vi "equilibrium_measurements.vi"() -> ()   [LabVIEW 2019]
uses:
  <vilib>/userDefined/High Color/IMAQdx.ctl
  <vilib>/vision/driver/IMAQdx.llb/IMAQdx Attribute Type.ctl
  <vilib>/vision/Management.llb/Cast Image 2 Method.ctl
  <vilib>/DAQmx/write.llb/DAQmx Write (Analog DBL 1Chan 1Samp).vi
  <vilib>/DAQmx/read.llb/DAQmx Read (Analog DBL 1Chan 1Samp).vi
  <vilib>/Analysis/baseanly.llb/Mean (DBL).vi
  <vilib>/DAQmx/create/channels.llb/DAQmx Create Channel (AO-Voltage-Basic).vi
  <vilib>/DAQmx/miscellaneous.llb/DAQmx Fill In Error Info.vi
  <vilib>/DAQmx/create/channels.llb/DAQmx Create Channel (AI-Temperature-Thermocouple).vi
  <vilib>/vision/driver/NI_Vision_Acquisition_Software.lvlib
  <resource>/objmgr/imaqdx.rc
  <vilib>/vision/NI_Vision_Development_Module.lvlib
  <vilib>/Analysis/NI_AALBase.lvlib
panel:
  out "Video":bool
  in  "Action":i32(listbox)
  out "meanIntensity":dbl[](array[numeric])
  out "varLaplacian":dbl[](array[numeric])
  out "mean":dbl
  out "variance":dbl
  out "Avg Intensity":dbl(graph)=4.716017316017316
  in  "Activate":bool
  out "Var of Laplacian":dbl(graph)=63.940469067936796
  out "Camera Display 2":T1(plugin-control) caption="Image Out"
  in  "ROI":T2={"Global Rectangle"=[], "Contours"=[{"Contour Type"=0, "ROI Type"=3, "Points"=[231, 86, 235, 90]}, {"Contour Type"=0, "ROI Type"=3, "Points"=[193, 50, 270, 125]}]}
  in  "error in":errorcluster
  in  "File path for video":string="C:\\Users\\Aniket\\Desktop\\mCherry_calibration\\new_lens\\laser_calibration\\laser_and_heating\\"
  in  "Laser profile file path":path=path "C:/Users/Aniket/Desktop/mCherry_calibration/new_lens/laser_calibration/laser_profiles/new_profile.txt"
  in  "Trigger Laser":bool
  in  "Power Generator":refnum<visa-resource-name>="COM3"
  in  "Desired \nTemperature":dbl=20.0 format="%#_13g"
  in  "PID Control":bool
  in  "Image file path \n(Do not add specify file extension - set to png)":path=path "C:/Users/Aniket/Desktop/mCherry_calibration/new_lens/laser_calibration/laser_profiles.txt"
  out "Current \nTemperature":dbl format="%0.2f"
  out "?":dbl[](graph)=[37.63236695538445]
  out "error out 7":errorcluster
  out "error out 6":errorcluster
  out "error out 5":errorcluster
  out "Exposure Time":dbl
  in  "ON/OFF":bool
  out "error out 3":errorcluster
  in  "LED":dbl(slide) scale=0.0..10.0
  in  "Refresh":bool
  out "Record":bool
  out "Processed Frames per Second":dbl
  out "Acquired Frame Rate":dbl
  out "error out":errorcluster
  out "Camera Display":T1(plugin-control) caption="Image Out"
  in  "Frame Rate":dbl=20.0
  out "Attribute Information Array":T4(array[cluster])
  in  "Session In":T5="cam0"
  # "Spot motion"
  # "Stage motion"
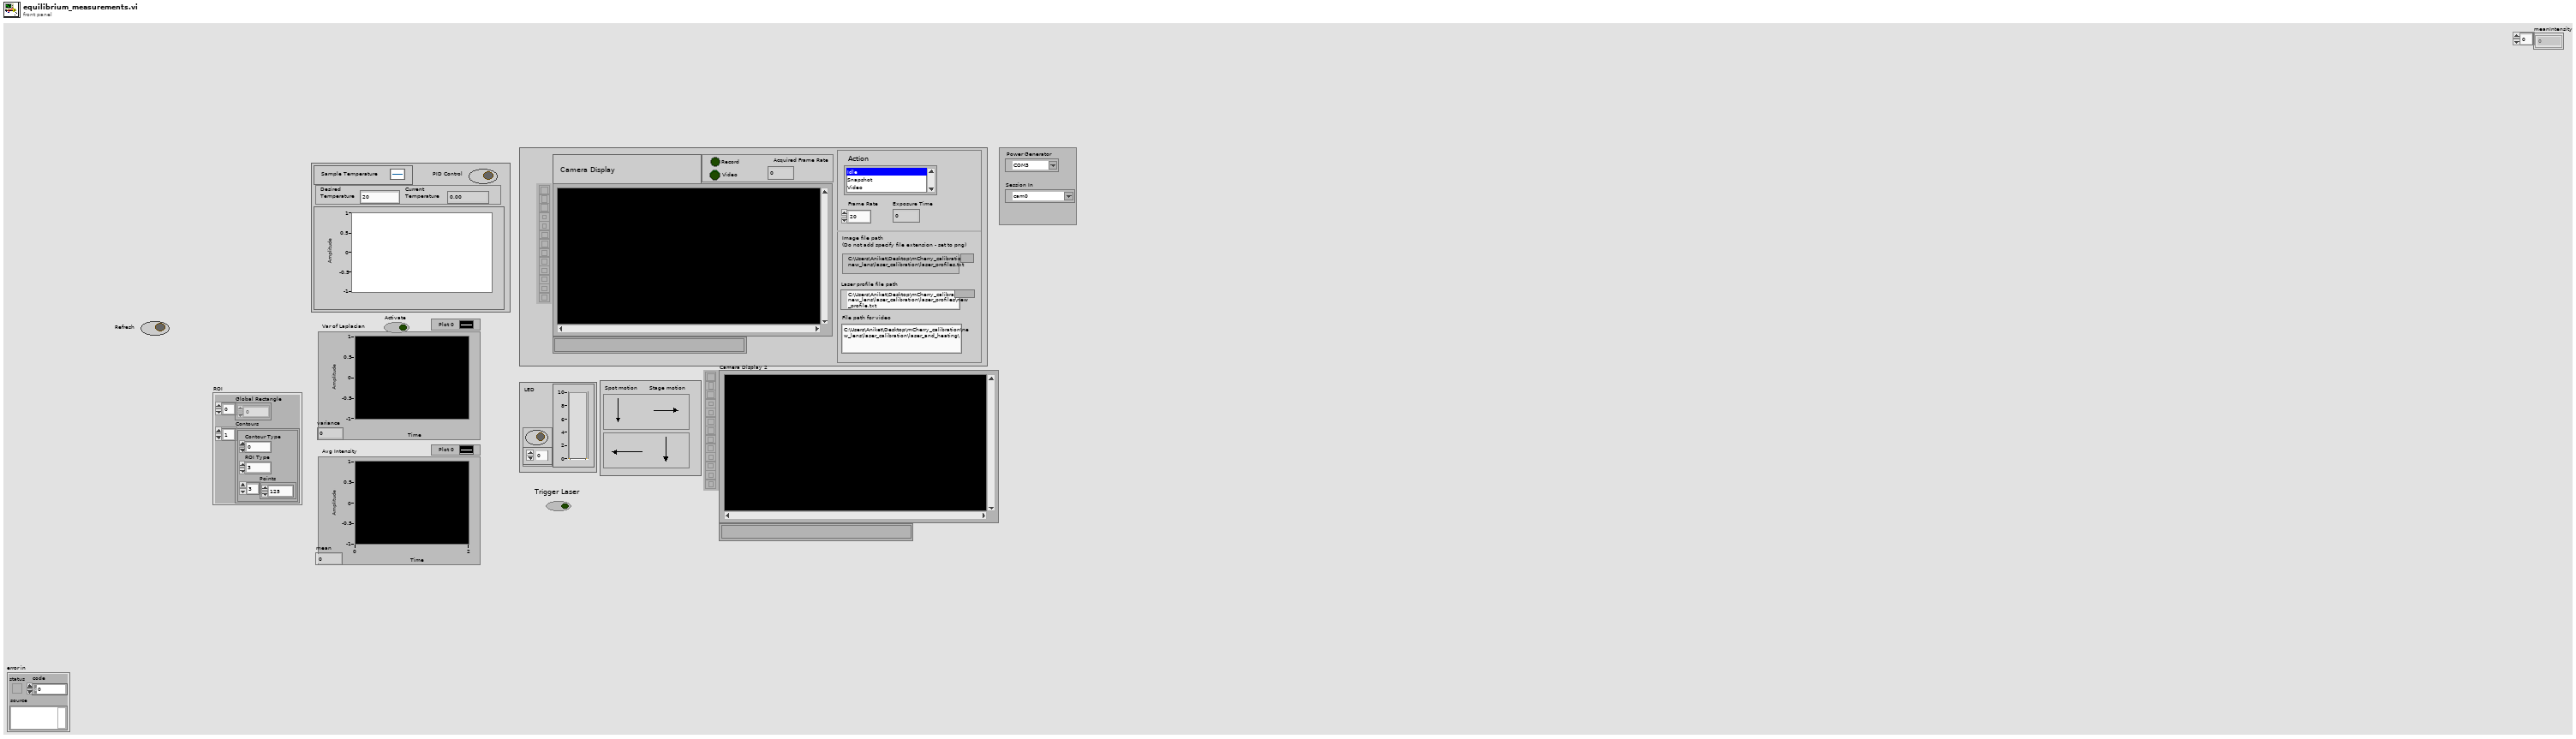
[diagram p1: front panel]
types:
  T1 = typedef "IMAQ Image.ctl" = refnum<image>
  T2 = cluster{"Global Rectangle":i32[], "Contours":cluster{"Contour Type":u32, "ROI Type":u32, "Points":i32[]}[]}
  T3 = typedef "NI_Vision_Acquisition_Software.lvlib/IMAQdx Attribute Type.ctl" = enum32{"U32", "I64", "DBL", "String", "Enum", "Bool", "Command"}
  T4 = cluster{"Attribute Type":T3, "Readable":bool, "Writable":bool, "Attribute Name":string}[]
  T5 = typedef "IMAQdx.ctl" = refnum<k21>
  T6 = typedef "Image Type" = u32
  T7 = typedef "ROI Descriptor" = cluster{"Global Rectangle":i32[], "Contours":cluster{"ID":enum32{"External", "Internal"}, "Type":u32, "Coordinates":i32[]}[]}
  T8 = typedef "IMAQ Rectangle" = cluster{"Left":i32, "Top":i32, "Right":i32, "Bottom":i32, "Rotation":dbl}
  T9 = typedef "Cast Image 2 Method.ctl" = u32
  T10 = typedef "IMAQ AVI2 Refnum.ctl" = refnum<k20>
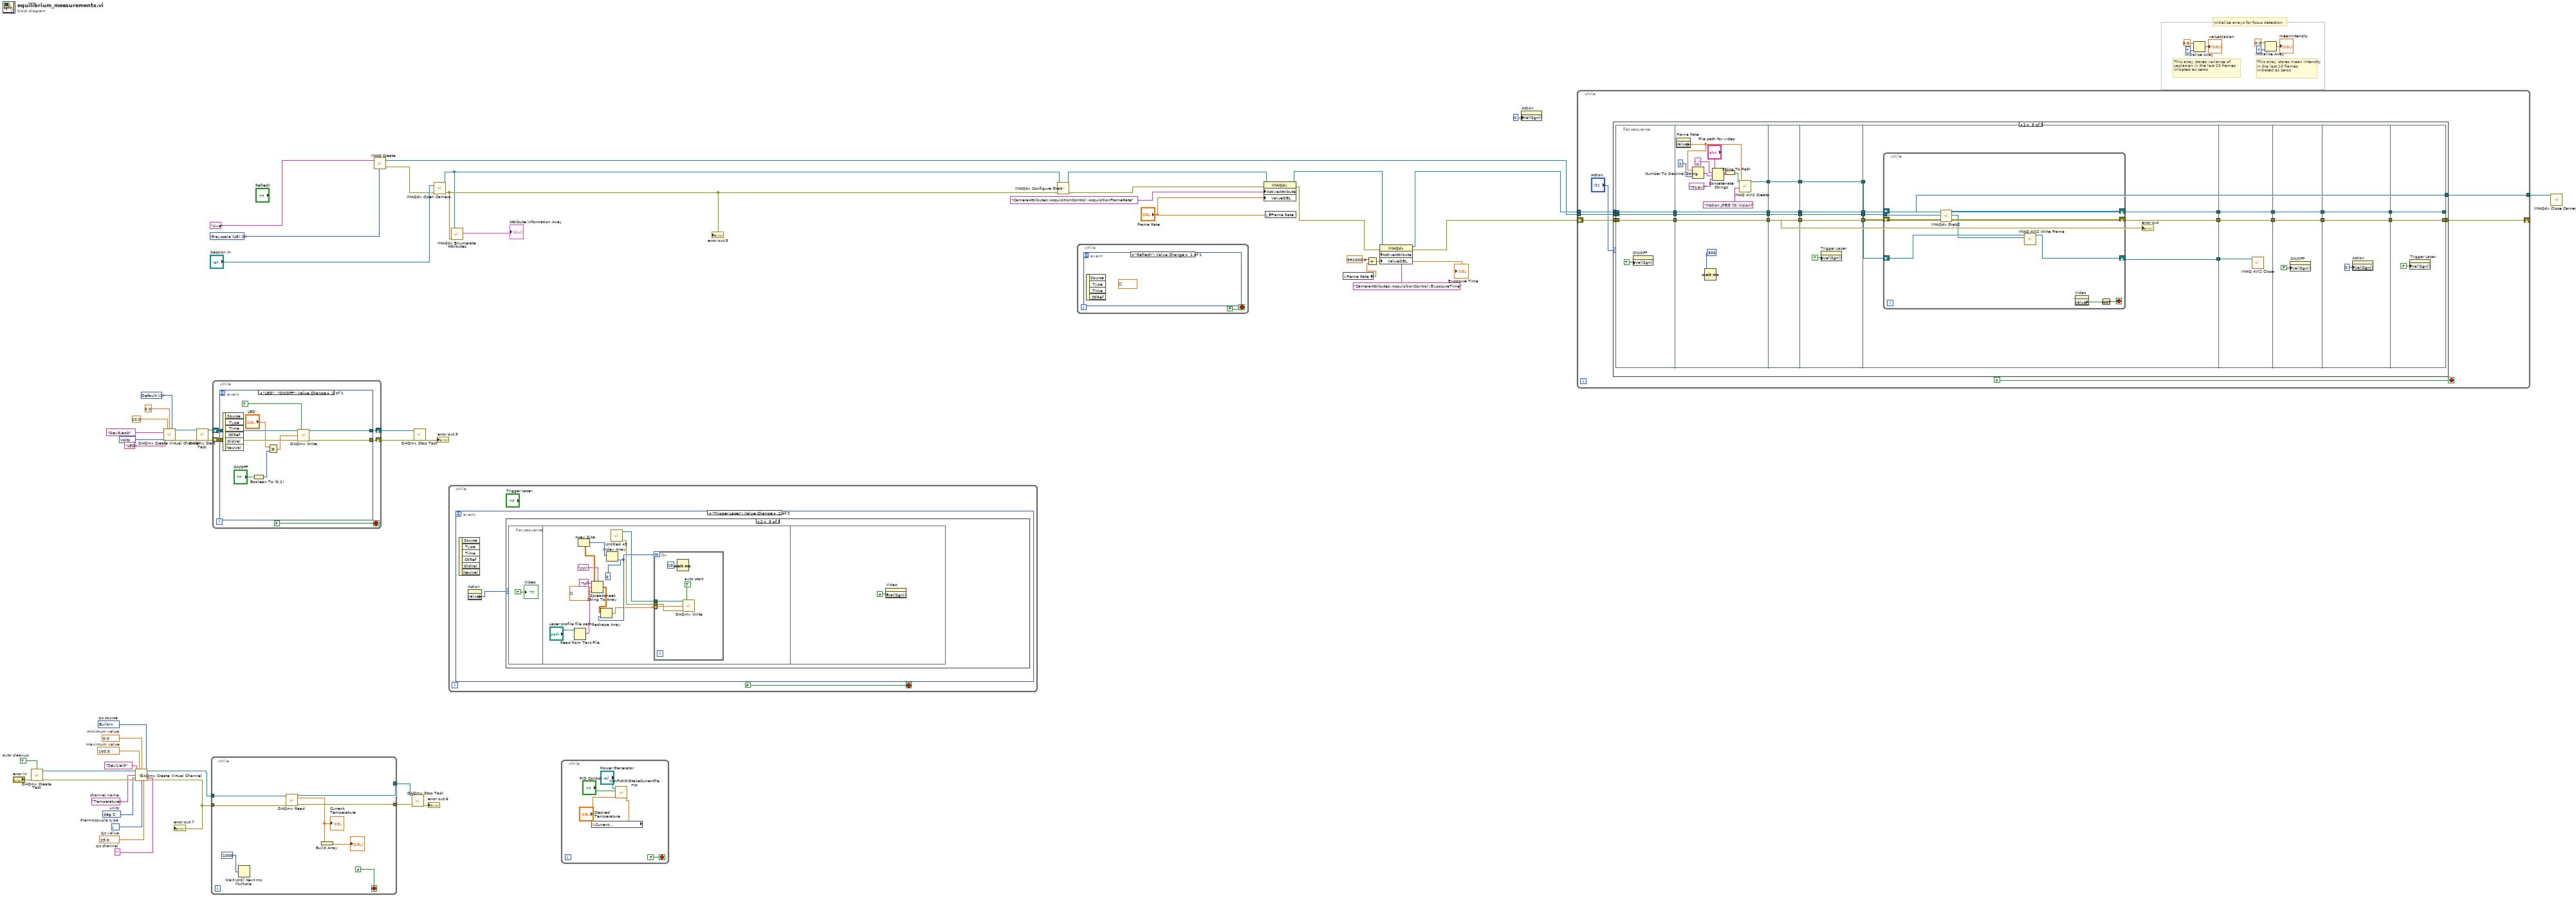
[diagram p0: block diagram]
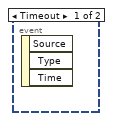
[diagram p2: hidden frame]
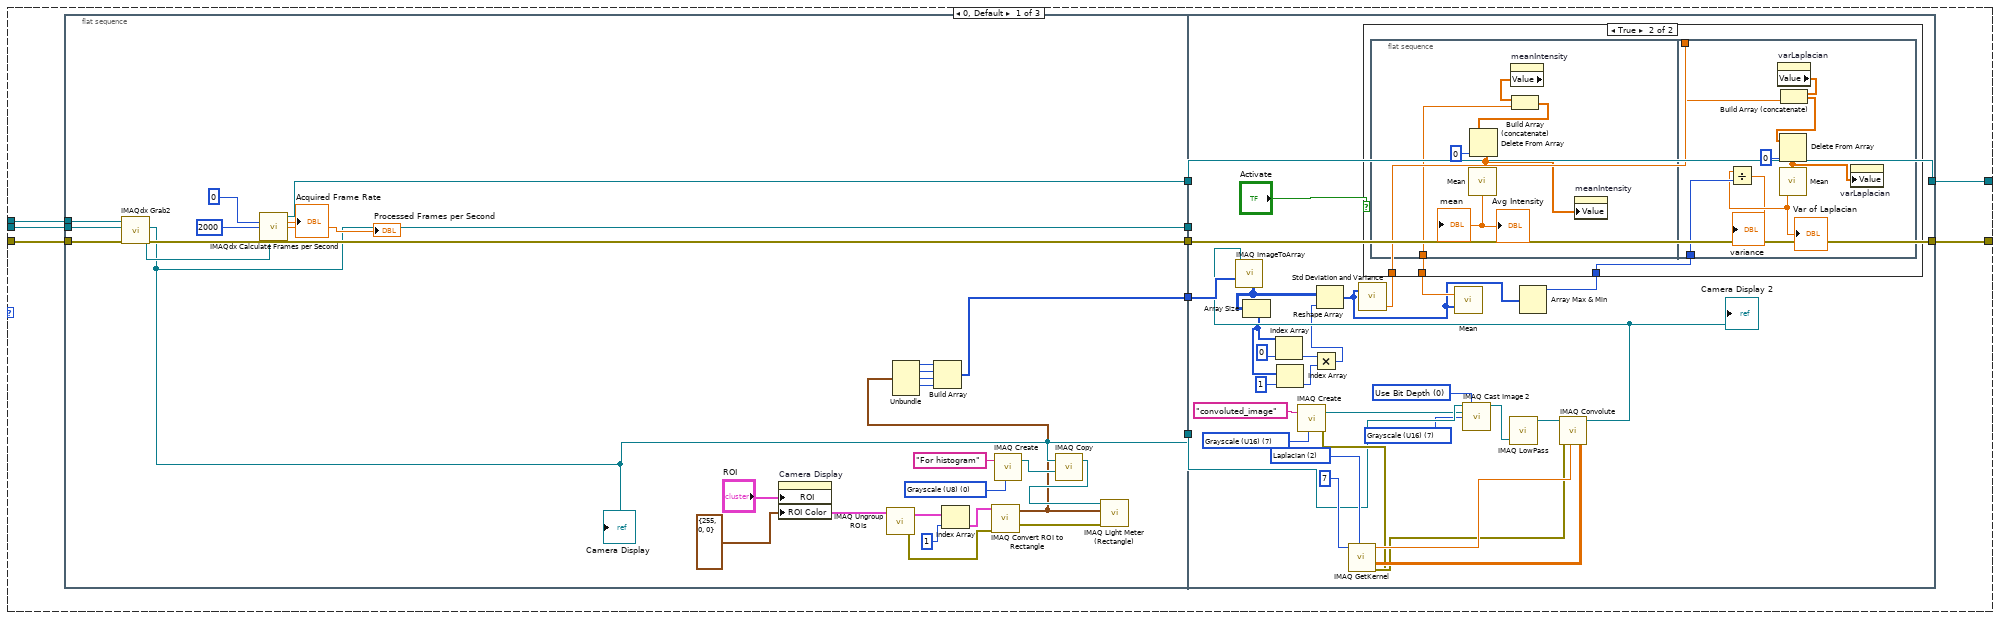
[diagram p5: hidden frame]
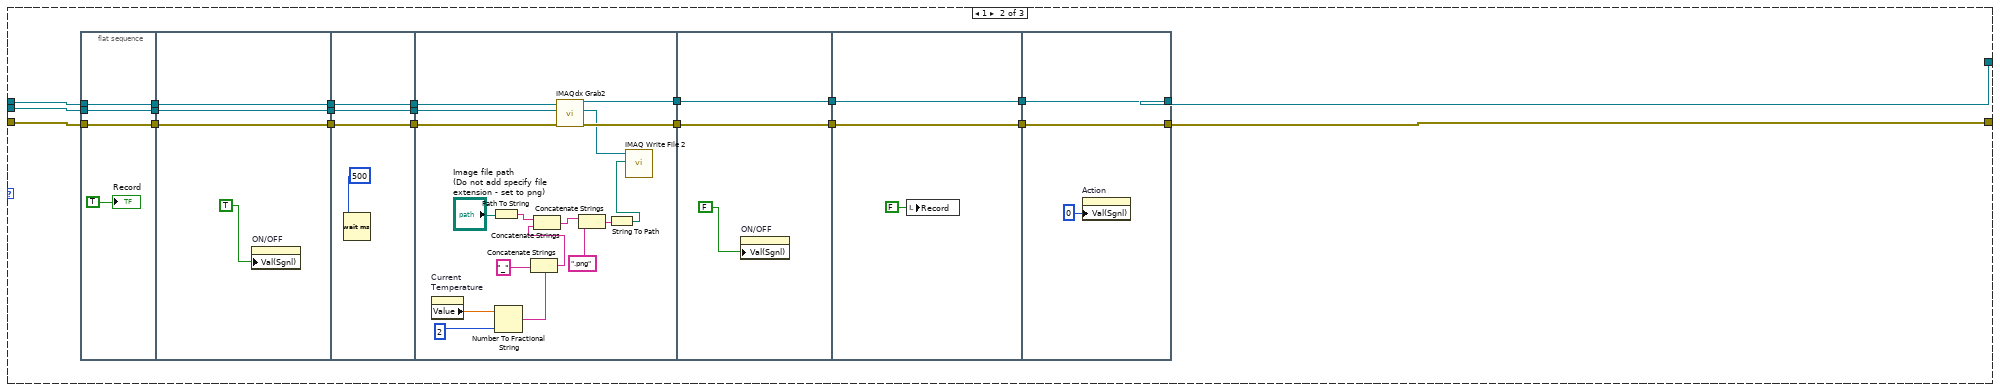
[diagram p7: hidden frame]
diagram:
  w12 = 10200 items=["Built-In"=10200, "Constant Value"=10116, "Channel"=10113]  # cjc source
  w14 = ""  # cjc channel
  w15 = 25.0  # cjc value
  w16 = 10072 items=["J"=10072, "K"=10073, "N"=10077, "R"=10082, "S"=10085, "T"=10086, "B"=10047, "E"=10055]  # thermocouple type
  w17 = 10143 items=["deg C"=10143, "deg F"=10144, "Kelvins"=10325, "deg R"=10145, "From Custom Scale"=10065]  # units
  w13 = "Temperature"  # channel name
  w18 = 0.0  # minimum value
  w19 = 100.0  # maximum value
  w21 = TRUE  # auto cleanup
  w44 = 10348 items=["Volts"=10348, "From Custom Scale"=10065] ("units")
  w46 = -1 items=["Default"=-1, "RSE"=10083, "NRSE"=10078, "Differential"=10106, "Pseudodifferential"=12529] ("input terminal configuration")
  w58 = T6 0 items=["Grayscale (U8)", "Grayscale (I16)", "Grayscale (SGL)", "Complex (CSG)", "RGB (U32)", "HSL (U32)", "RGB (U64)", "Grayscale (U16)"] ("Image Type")
  # "Initialize arrays for focus detection"
  # "This array stores mean intensity in the last 10 frames\nInitiated as zeros"
  # "This array stores variance of Laplacian in the last 10 frames\nInitiated as zeros"
  n1 = call <vilib>:"DAQmx Create Task.vi"("auto cleanup"=w21, "error in"="error in") -> ("task out"=w20:refnum<k21>, "error out"=w22:errorcluster)  [unwired: 12 in]
  n2 = call-poly <vilib>:"DAQmx Create Virtual Channel.vi"("task in"=w20, "maximum value"=w19, "minimum value"=w18, "physical channels"=tag "Dev1/ai0", "cjc source"=w12, "name to assign"=w13, "units"=w17, "cjc channel"=w14, "error in"=w22, "thermocouple type"=w16, "cjc value"=w15) -> ("task out"=w11:refnum<k21>, "error out"=w10:errorcluster)  [unwired: 3 in]
  "error out 7" <- w10
  n3 = call-poly <vilib>:"DAQmx Create Virtual Channel.vi"("maximum value"=10.0, "minimum value"=0.0, "output terminal configuration"=w46, "physical channels"=tag "Dev3/ao0", "name to assign"="LED", "units"=w44) -> ("task out"=w42:refnum<k21>, "error out"=w41:errorcluster)  [unwired: 8 in]
  n4 = call <vilib>:"DAQmx Start Task.vi"("task/channels in"=w42, "error in"=w41) -> ("task out"=w40:refnum<k21>, "error out"=w39:errorcluster)  [unwired: 12 in]
  n5 = while {
    tunnel: w11 -> [w67]
    tunnel: w10 -> [w66]
    tunnel: [w65] -> w26
    tunnel: [w64] -> w25
    stop <- FALSE ("Monitor Temperature") stop-if-true
    n6 = Wait Until Next ms Multiple(millisecond multiple=u32 1000 ("millisecond timer value")) -> ()  [unwired: 1 out]
    n7 = call-poly <vilib>:"DAQmx Read.vi"("task/channels in"=w67, "error in"=w66) -> ("task out"=w65:refnum<k21>, "data"=w61:dbl, "error out"=w64:errorcluster)  [unwired: 11 in]
    "Current \nTemperature" <- w61
    n8 = Build Array(w61) -> (→"?":dbl[])
  }
  n9 = while {
    shift-right: [w71] -> w38
    shift-left: w40 -> [w73]
    shift-right: [w70] -> w37
    shift-left: w39 -> [w72]
    stop <- FALSE stop-if-true
    n10 = event shown="[0] \"LED\", \"ON/OFF\": Value Change" {
      selector: _ -> [_]
      dyn-events: _ -> [_]
      timeout: _ -> [_]
      tunnel: w73 -> [w82]
      tunnel: w72 -> [w81]
      tunnel: [w80] -> w71
      tunnel: [w79] -> w70
      event "LED", "ON/OFF": Value Change {
        n11 = event-data() -> ()  [unwired: 1 in, 6 out]
        n12 = Boolean To (0,1)(Boolean="ON/OFF") -> (0, 1=w75:i16)
        n13 = Multiply(x="LED", y=w75) -> (x*y=w74:dbl)
        n14 = call-poly <vilib>:"DAQmx Write.vi"("task/channels in"=w82, "auto start"=TRUE, "data"=w74, "error in"=w81) -> ("task out"=w80:refnum<k21>, "error out"=w79:errorcluster)  [unwired: 9 in, 1 out]
      }
    }
  }
  n15 = call "IMAQ Create"("Image Name"="Live", "Image Type"=w58) -> ("New Image"=w52:T1, "error out"=w51:errorcluster)  [unwired: 3 in]
  n16 = call <vilib>:"DAQmx Stop Task.vi"("task/channels in"=w26, "error in"=w25) -> ("error out"=→"error out 6":errorcluster)  [unwired: 12 in, 1 out]
  n17 = call <vilib>:"DAQmx Stop Task.vi"("task/channels in"=w38, "error in"=w37) -> ("error out"=→"error out 3":errorcluster)  [unwired: 12 in, 1 out]
  n18 = call <vilib>:"IMAQdx Open Camera.vi"("error in"=w51, "Session In"="Session In") -> ("error out"=w56:errorcluster, "Session Out"=w57:T5)  [unwired: 8 in]
  "error out 5" <- w56
  n19 = while {
    stop <- FALSE stop-if-true
    n20 = event shown="[1] \"Trigger Laser\": Value Change" {
      selector: _ -> [_ _]
      dyn-events: _ -> [_ _]
      timeout: _ -> [_ _]
      event Timeout {
        n21 = event-data() -> ()  [unwired: 1 in, 3 out]
      }
      event "Trigger Laser": Value Change {
        n22 = event-data() -> ()  [unwired: 1 in, 6 out]
        n23 = property on="Action" class="LstBox (strict)"() -> ("Value"=w84:i32)  [unwired: 2 in, 2 out]
        n24 = case shown="2" w84 {
          frame 0, Default {
          }
          frame 1 {
          }
          frame 2 {
            n25 = flat-sequence {
              frame #0 {
                "Video" <- TRUE ("Video")
              }
              frame #1 {
                n26 = Read from Text File(file (use dialog)="Laser profile file path") -> (text=w93:string)  [unwired: 3 in, 3 out]
                n27 = Spreadsheet String To Array(delimiter (Tab)="\r\n", format string="%f", spreadsheet string=w93, array type (2D Dbl)=dbl[][] []) -> (array=w95:dbl[][])
                n28 = Array Size(array=w95) -> (size(s)=w94:i32[])
                n29 = Index Array(array=w94, index=0) -> (element=w97:i32)
                n30 = Reshape Array(w95, w97) -> (w96:dbl[])
                n31 = call "Untitled 43.vi"() -> ("error out"=w86:errorcluster, "task out"=w87:refnum<k21>)  [unwired: 10 in]
                n32 = for {
                  N: w97 -> [_]
                  tunnel: w96 -> [w98] mode=indexing
                  tunnel: w87 -> [w100]
                  tunnel: w86 -> [w99]
                  w101 = TRUE  # auto start
                  n33 = Wait (ms)(milliseconds to wait=u32 10) -> ()  [unwired: 1 out]
                  n34 = call-poly <vilib>:"DAQmx Write.vi"("task/channels in"=w100, "auto start"=w101, "data"=w98, "error in"=w99) -> ()  [unwired: 9 in, 3 out]
                }
              }
              frame #2 {
                n35 = property on="Video" class="Bool (strict)"("Val(Sgnl)"=FALSE ("Value (Signaling)")) -> ()  [unwired: 2 in, 2 out]
              }
            }
          }
        }
      }
    }
  }
  n36 = call <vilib>:"IMAQdx Enumerate Attributes.vi"("error in"=w56, "Session In"=w57) -> ("Attribute Information Array"=→"Attribute Information Array":T4)  [unwired: 7 in, 2 out]
  n37 = while {
    stop <- FALSE stop-if-true
    n38 = local read "Current \nTemperature"() -> (w106:dbl)
    n39 = call "IronFishPIDtakeCurrentTemp.vi"("Current Temp"=w106, "Desired Temp"="Desired \nTemperature", "Switch"="PID Control", 11:"Power Generator") -> ()  [unwired: 8 in]
  }
  n40 = call <vilib>:"IMAQdx Configure Grab.vi"("error in"=w56, "Session In"=w57) -> ("error out"=w54:errorcluster, "Session Out"=w35:T5)  [unwired: 8 in]
  n41 = while {
    stop <- FALSE stop-if-true
    n42 = event shown="[0] \"Refresh\": Value Change" {
      selector: _ -> [_]
      dyn-events: _ -> [_]
      timeout: _ -> [_]
      event "Refresh": Value Change {
        (unwired) dbl[] [] ("History Data")
        n43 = event-data() -> ()  [unwired: 1 in, 4 out]
      }
    }
  }
  n44 = property class="IMAQdx"(reference=w35, error in=w54, "ActiveAttribute"="CameraAttributes::AcquisitionControl::AcquisitionFrameRate", "ValueDBL"="Frame Rate") -> (reference out=w30:T5, error out=w28:errorcluster)
  n45 = local write "Frame Rate"("Frame Rate") -> ()
  n46 = local read "Frame Rate"() -> (w32:dbl)
  n47 = Divide(x=991000.0, y=w32) -> (x/y=w31:dbl)
  "Exposure Time" <- w31
  n48 = property class="IMAQdx"(reference=w30, error in=w28, "ActiveAttribute"="CameraAttributes::AcquisitionControl::ExposureTime", "ValueDBL"=w31) -> (reference out=w29:T5, error out=w27:errorcluster)
  n49 = property on="Action" class="LstBox (strict)"("Val(Sgnl)"=0 ("Value (Signaling)")) -> ()  [unwired: 2 in, 2 out]
  n50 = while {
    tunnel: w29 -> [w116]
    tunnel: w52 -> [w114]
    shift-right: [w113] -> w50
    shift-left: w27 -> [w115]
    tunnel: [w110] -> w2
    stop <- FALSE ("Stop") stop-if-true
    n51 = case shown="2" "Action" {
      tunnel: w116 -> [w126 w217 w288]
      tunnel: w115 -> [w125 w219 w286]
      tunnel: w114 -> [w124 w218 w287]
      tunnel: [w123 w220 w284] -> w113
      tunnel: [w122 w221 w285] -> w110
      frame 0, Default {
        n52 = flat-sequence {
          tunnel: w126 -> [w154]
          tunnel: w125 -> [w153]
          tunnel: w124 -> [w152]
          tunnel: [w151] -> w121
          tunnel: [w149] -> w120
          tunnel: [w136] -> w119
          tunnel: [w136] -> w118
          tunnel: [w128] -> w117
          tunnel: [w183] -> w122
          tunnel: [w184] -> w123
          tunnel: w121 -> [w184]
          tunnel: w120 -> [w183]
          tunnel: w119 -> [_]
          tunnel: w118 -> [w164]
          tunnel: w117 -> [w174]
          frame #0 {
            w137 = T6 0 items=["Grayscale (U8)", "Grayscale (I16)", "Grayscale (SGL)", "Complex (CSG)", "RGB (U32)", "HSL (U32)", "RGB (U64)", "Grayscale (U16)"] ("Image Type")
            n53 = call <vilib>:"IMAQdx Grab2.vi"("error in"=w153, "Image In"=w152, "Session In"=w154) -> ("error out"=w151:errorcluster, "Image Out"=w136:T1, "Session Out"=w150:T5)  [unwired: 5 in, 1 out]
            "Camera Display" <- w136
            n54 = call <vilib>:"IMAQdx Calculate Frames per Second.vi"("Session In"=w150, "Buffer Number"=u32 0, "Minimum Display Update Interval (ms)"=u32 2000) -> ("Session Out"=w149:T5, "Acquired Frames per Second"=→"Acquired Frame Rate":dbl, "Processed Frames per Second"=→"Processed Frames per Second":dbl)  [unwired: 6 in, 4 out]
            n55 = property on="Camera Display" class="ImageControl"("ROI"="ROI", "ROI Color"=cluster{"Red":u8, "Green":u8, "Blue":u8} {"Red"=255, "Green"=0, "Blue"=0}) -> ()  [unwired: 2 in, 2 out]
            n56 = call "IMAQ Ungroup ROIs"("ROI Descriptor"="ROI") -> ("error out"=w140:errorcluster, "ROI Descriptors out"=w143:T7[])  [unwired: 3 in]
            n57 = Index Array(array=w143, index=1) -> (element=w141:T7)
            n58 = call "IMAQ Convert ROI to Rectangle"("error in (no error)"=w140, "ROI Descriptor"=w141) -> ("error out"=w139:errorcluster, "Rectangle"=w133:T8)  [unwired: 7 in]
            n59 = Unbundle(w133) -> ("Left"=w132:i32, "Top"=w131:i32, "Right"=w130:i32, "Bottom"=w129:i32)  [unwired: 1 out]
            n60 = Build Array(w132, w131, w130, w129) -> (w128:i32[])
            n61 = call "IMAQ Create"("Image Name"="For histogram", "Image Type"=w137) -> ("New Image"=w135:T1)  [unwired: 3 in, 1 out]
            n62 = call "IMAQ Copy"("Image Dst"=w135, "Image Src"=w136) -> ("Image Dst Out"=w134:T1)  [unwired: 4 in, 1 out]
            n63 = call "IMAQ Light Meter (Rectangle)"("error in (no error)"=w139, "Rectangle"=w133, "Image"=w134) -> ()  [unwired: 4 in, 5 out]
          }
          frame #1 {
            w160 = T6 7 items=["Grayscale (U8)", "Grayscale (I16)", "Grayscale (SGL)", "Complex (CSG)", "RGB (U32)", "HSL (U32)", "RGB (U64)", "Grayscale (U16)"] ("Image Type")
            w163 = T9 0 items=["Use Bit Depth", "Shift", "Use Lookup Table"] ("Method")
            w179 = u16 2 items=["Gradient"=1, "Laplacian"=2, "Smoothing"=3, "Gaussian"=4] ("Kernel Family")
            w181 = T6 7 items=["Grayscale (U8)", "Grayscale (I16)", "Grayscale (SGL)", "Complex (CSG)", "RGB (U32)", "HSL (U32)", "RGB (U64)", "Grayscale (U16)"] ("Image Type")
            n64 = call "IMAQ Create"("Image Name"="convoluted_image", "Image Type"=w181) -> ("New Image"=w162:T1, "error out"=w175:errorcluster)  [unwired: 3 in]
            n65 = call "IMAQ GetKernel"("Kernel Family"=w179, "error in (no error)"=w175, "Kernel Size (3,5,...)"=7) -> ("error out"=w176:errorcluster, "Kernel"=w177:sgl[][], "Divider"=w178:sgl)  [unwired: 5 in, 1 out]
            n66 = call "IMAQ Cast Image 2"("Image Src"=w164, "Method"=w163, "Image Dst"=w162, "Image Type"=w160) -> ("Image Dst Out"=w161:T1)  [unwired: 10 in, 1 out]
            n67 = call "IMAQ LowPass"("Image Src"=w161) -> ("Image Dst Out"=w165:T1)  [unwired: 6 in, 1 out]
            n68 = call "IMAQ Convolute"("Kernel"=w177, "Divider (kernel sum)"=w178, "error in (no error)"=w176, "Image Src"=w165) -> ("Image Dst Out"=w173:T1)  [unwired: 6 in, 1 out]
            "Camera Display 2" <- w173
            n69 = call "IMAQ ImageToArray"("Optional Rectangle"=w174, "Image"=w173) -> ("Image Pixels (U16)"=w158:u16[][])  [unwired: 2 in, 4 out]
            n70 = Array Size(array=w158) -> (size(s)=w159:i32[])
            n71 = Index Array(array=w159, index=0 ("index (row)")) -> (element=w170:i32)
            n72 = Index Array(array=w159, index=1) -> (element=w169:i32)
            n73 = Multiply(x=w170, y=w169) -> (x*y=w157:i32)
            n74 = Reshape Array(w158, w157) -> (w156:u16[])
            n75 = call <vilib>:"Std Deviation and Variance.vi"("X"=w156) -> ("variance"=w167:dbl)  [unwired: 1 in, 2 out]
            n76 = call-poly <vilib>:"Mean.vi"("X"=w156) -> ("mean"=w166:dbl)  [unwired: 1 out]
            n77 = Array Max & Min(array=w156) -> (max value=w155:u16)  [unwired: 3 out]
            n78 = case shown="True" "Activate" {
              tunnel: w167 -> [_ w186]
              tunnel: w166 -> [_ w187]
              tunnel: w155 -> [_ w185]
              frame False {
              }
              frame True {
                n79 = flat-sequence {
                  tunnel: w187 -> [w190]
                  tunnel: w186 -> [w196]
                  tunnel: w185 -> [w201]
                  frame #0 {
                    n80 = property on="meanIntensity" class="Arr (strict)"() -> ("Value"=w191:dbl[])  [unwired: 2 in, 2 out]
                    n81 = Build Array (concatenate)(w191, w190) -> (w189:dbl[])
                    n82 = Delete From Array(array=w189, index=0) -> (array with subset deleted=w188:dbl[])  [unwired: 1 in, 1 out]
                    n83 = call-poly <vilib>:"Mean.vi"("X"=w188) -> ("mean"=→"Avg Intensity" →"mean":dbl)  [unwired: 1 out]
                    n84 = property on="meanIntensity" class="Arr (strict)"("Value"=w188) -> ()  [unwired: 2 in, 2 out]
                  }
                  frame #1 {
                    n85 = property on="varLaplacian" class="Arr (strict)"() -> ("Value"=w197:dbl[])  [unwired: 2 in, 2 out]
                    n86 = Build Array (concatenate)(w197, w196) -> (w195:dbl[])
                    n87 = Delete From Array(array=w195, index=0) -> (array with subset deleted=w194:dbl[])  [unwired: 1 in, 1 out]
                    n88 = call-poly <vilib>:"Mean.vi"("X"=w194) -> ("mean"=w200:dbl)  [unwired: 1 out]
                    "Var of Laplacian" <- w200
                    n89 = Divide(x=w200, y=w201) -> (x/y=→"variance":dbl)
                    n90 = property on="varLaplacian" class="Arr (strict)"("Value"=w194) -> ()  [unwired: 2 in, 2 out]
                  }
                }
              }
            }
          }
        }
      }
      frame 1 {
        n91 = flat-sequence {
          tunnel: w217 -> [w223]
          tunnel: w218 -> [w224]
          tunnel: w219 -> [w225]
          tunnel: [w225] -> w206
          tunnel: [w224] -> w205
          tunnel: [w223] -> w204
          tunnel: [w229] -> w212
          tunnel: [w228] -> w210
          tunnel: [w227] -> w208
          tunnel: w206 -> [w229]
          tunnel: w205 -> [w228]
          tunnel: w204 -> [w227]
          tunnel: w212 -> [w233]
          tunnel: [w233] -> w211
          tunnel: w210 -> [w232]
          tunnel: [w232] -> w209
          tunnel: w208 -> [w231]
          tunnel: [w231] -> w207
          tunnel: [w246] -> w216
          tunnel: [w250] -> w214
          tunnel: w211 -> [w249]
          tunnel: w209 -> [w248]
          tunnel: w207 -> [w247]
          tunnel: w216 -> [w253]
          tunnel: [w253] -> w215
          tunnel: w214 -> [w252]
          tunnel: [w252] -> w213
          tunnel: w215 -> [w256]
          tunnel: w213 -> [w255]
          tunnel: [w256] -> w203
          tunnel: [w255] -> w202
          tunnel: [w258] -> w220
          tunnel: [w259] -> w221
          tunnel: w203 -> [w259]
          tunnel: w202 -> [w258]
          frame #0 {
            "Record" <- TRUE ("Record")
          }
          frame #1 {
            n92 = property on="ON/OFF" class="Bool (strict)"("Val(Sgnl)"=TRUE ("ON/OFF")) -> ()  [unwired: 2 in, 2 out]
          }
          frame #2 {
            n93 = Wait (ms)(milliseconds to wait=u32 500) -> ()  [unwired: 1 out]
          }
          frame #3 {
            n94 = property on="Current \nTemperature" class="DigNum (strict)"() -> ("Value"=w244:dbl)  [unwired: 2 in, 2 out]
            n95 = Path To String(path="Image file path \n(Do not add specify file extension - set to png)") -> (string=w239:string)
            n96 = Number To Fractional String(number=w244, precision (6)=i16 2 ("width (-)")) -> (F-format string=w241:string)  [unwired: 2 in]
            n97 = Concatenate Strings("_" ("string"), w241) -> (w238:string)
            n98 = Concatenate Strings(w239, w238) -> (w237:string)
            n99 = call <vilib>:"IMAQdx Grab2.vi"("error in"=w249, "Image In"=w248, "Session In"=w247) -> ("error out"=w250:errorcluster, "Image Out"=w245:T1, "Session Out"=w246:T5)  [unwired: 5 in, 1 out]
            n100 = Concatenate Strings(w237, ".png" ("string")) -> (w235:string)
            n101 = String To Path(string=w235) -> (path=w234:path)
            n102 = call-poly "IMAQ Write File 2"("File Path"=w234, "Image"=w245) -> ()  [unwired: 8 in, 2 out]
          }
          frame #4 {
            n103 = property on="ON/OFF" class="Bool (strict)"("Val(Sgnl)"=FALSE ("ON/OFF")) -> ()  [unwired: 2 in, 2 out]
          }
          frame #5 {
            n104 = local write "Record"(FALSE ("Record")) -> ()
          }
          frame #6 {
            n105 = property on="Action" class="LstBox (strict)"("Val(Sgnl)"=0 ("Value (Signaling)")) -> ()  [unwired: 2 in, 2 out]
          }
        }
      }
      frame 2 {
        n106 = flat-sequence {
          tunnel: w286 -> [w290]
          tunnel: w287 -> [w291]
          tunnel: w288 -> [w292]
          tunnel: [w292] -> w283
          tunnel: [w291] -> w282
          tunnel: [w290] -> w281
          tunnel: w283 -> [w306]
          tunnel: [w306] -> w280
          tunnel: w282 -> [w305]
          tunnel: [w305] -> w278
          tunnel: w281 -> [w304]
          tunnel: [w304] -> w276
          tunnel: [w301] -> w269
          tunnel: w280 -> [w310]
          tunnel: [w310] -> w279
          tunnel: w278 -> [w309]
          tunnel: [w309] -> w277
          tunnel: w276 -> [w308]
          tunnel: [w308] -> w275
          tunnel: [w307] -> w270
          tunnel: w269 -> [w307]
          tunnel: w279 -> [w312]
          tunnel: w277 -> [w313]
          tunnel: w275 -> [w314]
          tunnel: [w314] -> w274
          tunnel: [w313] -> w273
          tunnel: [w312] -> w272
          tunnel: [w311] -> w271
          tunnel: w270 -> [w311]
          tunnel: w274 -> [w321]
          tunnel: w273 -> [w320]
          tunnel: w272 -> [w319]
          tunnel: [w317] -> w268
          tunnel: [w318] -> w267
          tunnel: [w322] -> w266
          tunnel: w271 -> [w316]
          tunnel: w268 -> [w335]
          tunnel: [w335] -> w263
          tunnel: w267 -> [w334]
          tunnel: [w334] -> w265
          tunnel: w266 -> [w333]
          tunnel: w265 -> [w338]
          tunnel: [w338] -> w264
          tunnel: w263 -> [w337]
          tunnel: [w337] -> w262
          tunnel: w264 -> [w340]
          tunnel: w262 -> [w341]
          tunnel: [w341] -> w261
          tunnel: [w340] -> w260
          tunnel: [w343] -> w284
          tunnel: [w344] -> w285
          tunnel: w261 -> [w344]
          tunnel: w260 -> [w343]
          frame #0 {
            n107 = property on="ON/OFF" class="Bool (strict)"("Val(Sgnl)"=TRUE ("Value (Signaling)")) -> ()  [unwired: 2 in, 2 out]
          }
          frame #1 {
            n108 = property on="Frame Rate" class="DigNum (strict)"() -> ("Value"=w299:dbl)  [unwired: 2 in, 2 out]
            n109 = Number To Decimal String(number=w299, width (-)=i16 2) -> (decimal integer string=w294:string)
            n110 = Wait (ms)(milliseconds to wait=u32 500) -> ()  [unwired: 1 out]
            n111 = Concatenate Strings("File path for video", "_" ("string"), w294, "Hz.avi" ("string")) -> (w296:string)
            n112 = String To Path(string=w296) -> (path=w297:path)
            n113 = call "IMAQ AVI2 Create"("Codec"="Motion JPEG (NI Vision)", "Frames Per Second"=w299, "AVI Path"=w297) -> ("AVI Refnum"=w301:T10)  [unwired: 7 in, 1 out]
          }
          frame #2 {
          }
          frame #3 {
            n114 = property on="Trigger Laser" class="Bool (strict)"("Val(Sgnl)"=TRUE ("Value (Signaling)")) -> ()  [unwired: 2 in, 2 out]
          }
          frame #4 {
            n115 = while {
              tunnel: w320 -> [w330]
              shift-right: [w328] -> w318
              shift-left: w321 -> [w331]
              shift-right: [w327] -> w317
              shift-left: w319 -> [w329]
              shift-right: [w332] -> w322
              shift-left: w316 -> [w326]
              stop <- w324 stop-if-true
              n116 = call <vilib>:"IMAQdx Grab2.vi"("error in"=w331, "Image In"=w330, "Session In"=w329) -> ("error out"=w328:errorcluster, "Image Out"=w325:T1, "Session Out"=w327:T5)  [unwired: 5 in, 1 out]
              n117 = call "IMAQ AVI2 Write Frame"("Image"=w325, "AVI Refnum"=w326) -> ("AVI Refnum (duplicate)"=w332:T10)  [unwired: 7 in, 2 out]
              n118 = property on="Video" class="Bool (strict)"() -> ("Value"=w323:bool)  [unwired: 2 in, 2 out]
              n119 = Not(x=w323) -> (.not. x?=w324:bool)
            }
          }
          frame #5 {
            n120 = call "IMAQ AVI2 Close"("AVI Refnum"=w333) -> ()  [unwired: 10 in, 1 out]
          }
          frame #6 {
            n121 = property on="ON/OFF" class="Bool (strict)"("Val(Sgnl)"=FALSE ("Value (Signaling)")) -> ()  [unwired: 2 in, 2 out]
          }
          frame #7 {
            n122 = property on="Action" class="LstBox (strict)"("Val(Sgnl)"=0 ("Value (Signaling)")) -> ()  [unwired: 2 in, 2 out]
          }
          frame #8 {
            n123 = property on="Trigger Laser" class="Bool (strict)"("Val(Sgnl)"=FALSE ("Value (Signaling)")) -> ()  [unwired: 2 in, 2 out]
          }
        }
      }
    }
  }
  "error out" <- w50
  n124 = Initialize Array(0.0 ("element"), 7 ("dimension size")) -> (→"varLaplacian":dbl[])
  n125 = Initialize Array(0.0 ("element"), 7 ("dimension size")) -> (→"meanIntensity":dbl[])
  n126 = call <vilib>:"IMAQdx Close Camera.vi"("Session In"=w2) -> ()  [unwired: 10 in, 1 out]
